vi "CLSUIP_FindInterfacesInheritedByAncestor.vi"(11 "class":refnum<vi>) -> (3 "indirectly inherited interface item IDs":set{string}(c389))   [LabVIEW 2021]
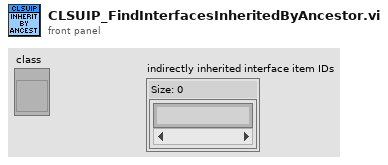
[diagram p1: front panel]
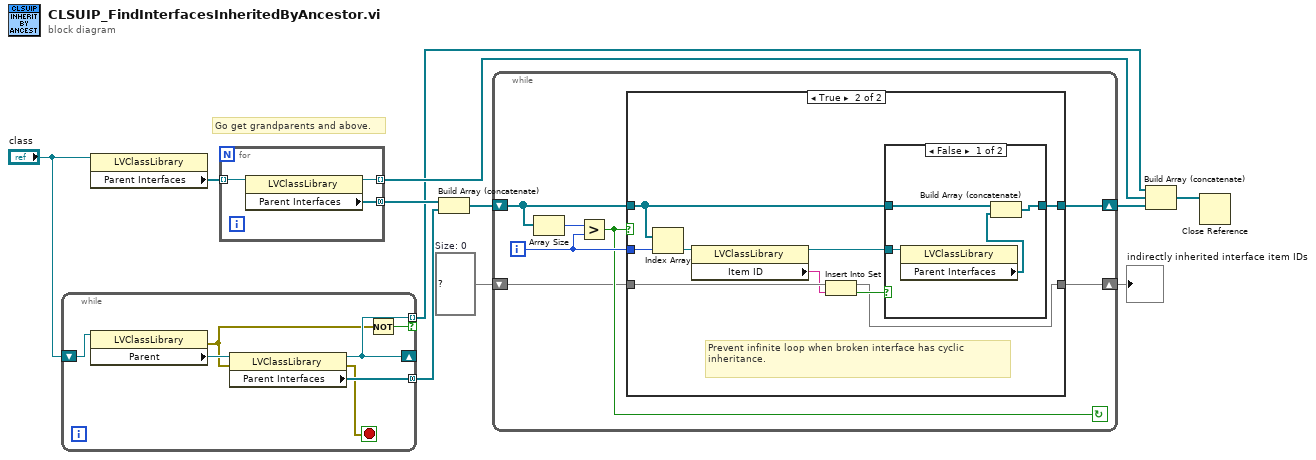
[diagram p0: block diagram]
diagram:
  w2 = set{string} {}  # Size: 0
  # "Go get grandparents and above."
  n1 = while {
    tunnel: [w17] -> w5 mode=concatenating
    shift-right: [w15] -> _
    shift-left: "class" -> [w18]
    tunnel: [w15] -> w3 mode=indexing if=w14
    stop <- w13 stop-if-true
    n2 = property class="LVClassLibrary"(reference=w18) -> (error out=w12:errorcluster, "Parent"=w16:refnum<vi>)  [unwired: 1 in, 1 out]
    n3 = property class="LVClassLibrary"(reference=w16, error in=w12) -> (reference out=w15:refnum<vi>, error out=w13:errorcluster, "Parent Interfaces"=w17:refnum<vi>[])
    n4 = Not(x=w12) -> (.not. x?=w14:bool)
  }
  n5 = property class="LVClassLibrary"(reference="class") -> ("Parent Interfaces"=w11:refnum<vi>[])  [unwired: 1 in, 2 out]
  n6 = for {
    tunnel: w11 -> [w21] mode=indexing
    tunnel: [w20] -> w6 mode=concatenating
    tunnel: [w19] -> w9 mode=indexing
    n7 = property class="LVClassLibrary"(reference=w21) -> (reference out=w19:refnum<vi>, "Parent Interfaces"=w20:refnum<vi>[])  [unwired: 1 in, 1 out]
  }
  n8 = Build Array (concatenate)(w6, w5) -> (w4:refnum<vi>[])
  n9 = while {
    shift-right: [w28] -> w10
    shift-left: w4 -> [w27]
    shift-right: [w22] -> w1
    shift-left: w2 -> [w23]
    i -> [w25]
    stop <- w24 continue-if-true
    n10 = Array Size(array=w27) -> (size(s)=w26:i32)
    n11 = Greater?(x=w26, y=w25) -> (0:w24:bool)
    n12 = case shown="True" w24 {
      tunnel: [w30 w39] -> w28
      tunnel: [w29 w32] -> w22
      tunnel: w27 -> [w30 w38]
      tunnel: w25 -> [_ w37]
      tunnel: w23 -> [w29 w35]
      frame False {
      }
      frame True {
        # "Prevent infinite loop when broken interface has cyclic inheritance."
        n13 = Index Array(array=w38, index=w37) -> (element=w36:refnum<vi>)
        n14 = property class="LVClassLibrary"(reference=w36) -> (reference out=w31:refnum<vi>, "Item ID"=w34:string)  [unwired: 1 in, 1 out]
        n15 = Insert Into Set(10:w34, 11:w35) -> (2:w33:bool, 3:w32:set{string})
        n16 = case shown="False" w33 {
          tunnel: [w43 w44] -> w39
          tunnel: w38 -> [w42 w44]
          tunnel: w31 -> [w41 _]
          frame False {
            n17 = property class="LVClassLibrary"(reference=w41) -> ("Parent Interfaces"=w40:refnum<vi>[])  [unwired: 1 in, 2 out]
            n18 = Build Array (concatenate)(w42, w40) -> (w43:refnum<vi>[])
          }
          frame True {
          }
        }
      }
    }
  }
  "indirectly inherited interface item IDs" <- w1
  n19 = Build Array (concatenate)(w3, w9, w10) -> (w8:refnum<vi>[])
  n20 = Close Reference(reference=w8) -> ()  [unwired: 1 in, 1 out]
